vi "get gran pH.vi"(8 "prev":T3 {"Va" format="%.2f"; "temperature" format="%.2f"; "channel 2" format="%.2f"; "channel 1" format="%.2f"}, 9 "sample":cluster{"Vo":dbl, "Na":dbl, "Measuring":bool} {"Na" format="%.4f"; "Vo" format="%.3f"}, 10 "min points":u8, 11 "Serial Port":refnum<visa-resource-name>) -> (0 "current":T3 {"Va" format="%.2f"; "temperature" format="%.2f"; "channel 2" format="%.2f"; "channel 1" format="%.2f"}, 1 "Gran plot":T1={"F1"=[], "Va"=[], "Ve"=0.5, "NC"=0.5, "r"=0.5, "Gran Plot"=[], "Measuring"=FALSE} {"r" format="%.4f"; "NC" format="%.3p"; "Ve" format="%.3f"; "Va" format="%.5f"; "F1" format="%.7f"}, 2 "Sample ID":u16, 3 "Serial Port out":refnum<visa-resource-name>, 4 "done":bool)   [LabVIEW 2010]
panel:
  in  "sensitivity":dbl=2.0 min=1.0 max=3.0 step=0.01 format="%.2f"
  in  "stop":bool
  in  "init gran":T2 {"time (s)" format="%.2f"; "temperature" format="%.2f"; "channel 2" format="%.2f"; "channel 1" format="%.2f"}
  out "pH":cluster{"time (s)":sgl[], "channel 1":dbl[]}(graph)
  out "Sample ID":u16
  out "current pH":dbl format="%.3f"
  in  "accept":bool
  in  "amount of titrant added":dbl format="%.2f"
  # "mL"
  # "accept pH value"
  # "end titration"
  # "F1 vs. Titrant volume"
  # "mL"
  # "eq/L"
  # "titrant volume"
  # "Normality of titrant"
  # "eq/L"
  # "mL"
  # "Volume of sample"
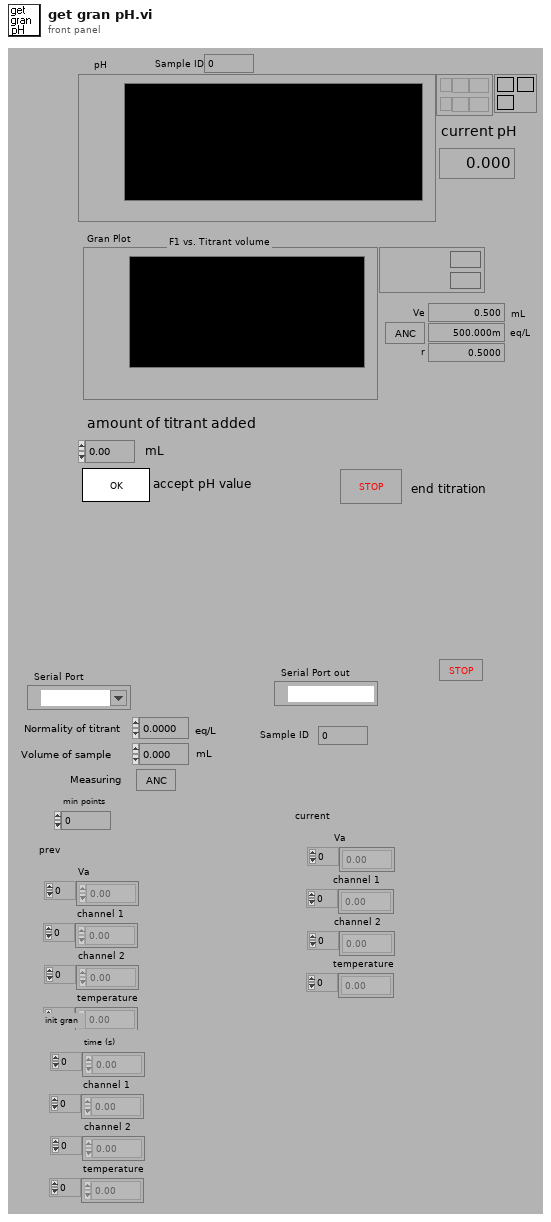
[diagram p1: front panel]
types:
  T1 = cluster{"F1":dbl[], "Va":dbl[], "Ve":dbl, "NC":dbl, "r":dbl, "Gran Plot":cluster{"Alkalinity":dbl[], "F1":dbl[]}[], "Measuring":bool}
  T2 = cluster{"channel 1":dbl[], "channel 2":dbl[], "temperature":dbl[], "time (s)":dbl[]}
  T3 = cluster{"channel 1":dbl[], "channel 2":dbl[], "temperature":dbl[], "Va":dbl[]}
  T4 = cluster{"channel 1":dbl[], "channel 2":dbl[], "temperature":dbl[], "time (s)":sgl[]}
  T5 = cluster{"F1":dbl[], "Va":dbl[], "Ve":dbl, "Alkalinity":dbl, "r":dbl, "graph":cluster{"Va":dbl[], "F1":dbl[]}[], "Measuring":bool}
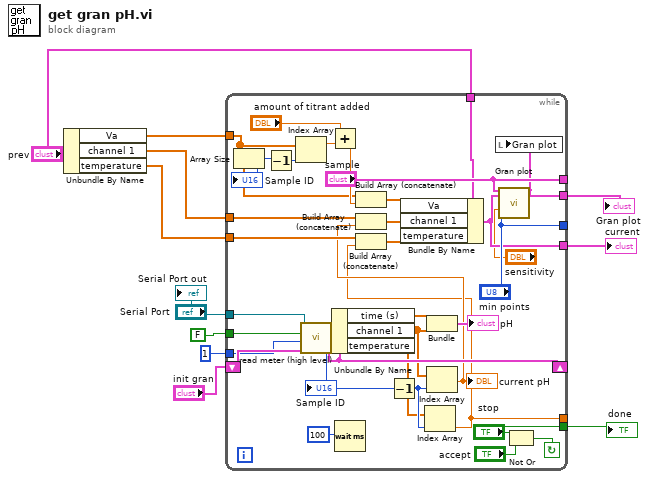
[diagram p0: block diagram]
diagram:
  n1 = Unbundle By Name("prev") -> ("Va"=w5:dbl[], "channel 1"=w4:dbl[], "temperature"=w3:dbl[])
  n2 = while {
    tunnel: "prev" -> [w13]
    tunnel: [w14] -> w1
    tunnel: [w15] -> w2
    tunnel: w3 -> [w21]
    tunnel: w4 -> [w22]
    tunnel: w5 -> [w24]
    tunnel: ["min points"] -> _
    tunnel: ["sample"] -> _
    tunnel: ["stop"] -> w6
    tunnel: [w16] -> _
    tunnel: 1 -> [w38]
    tunnel: FALSE -> [w39]
    tunnel: "Serial Port" -> [w40]
    shift-left: "init gran" -> [w45]
    shift-right: [w44] -> _
    stop <- w32 continue-if-true
    n3 = Array Size(array=w24) -> (size(s)=w25:i32)
    "Sample ID" <- w25
    n4 = Decrement(x=w25) -> (x-1=w26:i32)
    n5 = Index Array(array=w24, index=w26) -> (element=w27:dbl)
    n6 = call "read meter (high level).vi"("previous values"=w45, "seconds/data point"=w38, "2nd channel"=w39, "Serial Port"=w40) -> ("current values"=w44:T4, "Sample ID"=w42:u16)  [unwired: 2 in, 4 out]
    "Sample ID" <- w42
    n7 = Add(x="amount of titrant added", y=w27) -> (x+y=w28:dbl)
    n8 = Unbundle By Name(w44) -> ("time (s)"=w41:sgl[], "channel 1"=w37:dbl[], "temperature"=w35:dbl[])
    n9 = Wait (ms)(milliseconds to wait=100) -> ()  [unwired: 1 out]
    n10 = Build Array (concatenate)(w24, w28) -> (w20:dbl[])
    n11 = Decrement(x=w42) -> (x-1=w36:u16)
    n12 = Index Array(array=w35, index=w36) -> (element=w16:dbl)
    n13 = Build Array (concatenate)(w21, w16) -> (w18:dbl[])
    n14 = Bundle("time (s)"=w41, "channel 1"=w37) -> (→"pH":cluster{"time (s)":sgl[], "channel 1":dbl[]})  [unwired: 1 in]
    n15 = Index Array(array=w37, index=w36) -> (element=w17:dbl)
    "current pH" <- w17
    n16 = Build Array (concatenate)(w22, w17) -> (w19:dbl[])
    n17 = Bundle By Name(cluster=w13, "Va"=w20, "channel 1"=w19, "temperature"=w18) -> (w14:T3)
    n18 = call "Gran plot.vi"("sample"="sample", "current"=w14, "sensitivity"="sensitivity", "min points"="min points") -> ("Gran plot"=w15:T5)  [unwired: 11 in]
    n19 = local write "Gran plot"(w15) -> ()
    n20 = Not Or(1:"accept", 2:"stop") -> (0:w32:bool)
  }
  "current" <- w1
  "done" <- w6
  "Gran plot" <- w2
  "Serial Port out" <- "Serial Port"
